vi "integracao_1.03.vi"() -> ()   [LabVIEW 2011]
panel:
  out "Waveform Chart 4":dynamicdata(graph)
  out "Waveform Chart 3":dbl(graph)
  in  "Numeric 7":dbl
  in  "Numeric 6":dbl
  in  "Numeric 5":dbl
  in  "Numeric 4":dbl
  in  "Numeric 3":dbl
  in  "Numeric 2":dbl
  in  "Numeric":dbl
  in  "tail n-1":dbl
  in  "tail":dbl
  out "Integral 2 anter":dbl
  out "Integral 2 n-1":dbl
  out "Area  pico":dbl
  out "tempo 3":dbl
  out "Integral 3":dbl
  out "slope neg n-1":bool
  out "tempo 2":dbl
  out "Integral 2":dbl
  out "slope pos n-1":bool
  in  "picos":dbl
  out "Boolean 4":bool
  out "appended path":path
  out "String":string
  in  "Arquivo de entrada 2":path=path "C:/Works/GC3000/datalog/GC3000"
  out "Array":string[](array[string])
  out "Integral":dbl
  out "pico real":bool
  out "slope negativo":bool
  out "slope positivo":bool
  out "delta tempo menor 0,025":bool
  out "sinal menor que 1":bool
  out "signal 2":dbl
  out "Boolean 3":bool
  out "tempo":dbl
  out "Boolean 2":bool
  out "Waveform Chart 2":dynamicdata(graph)
  out "Boolean":bool
  out "slop curve":dbl
  out "Result":dbl
  out "signal":dbl
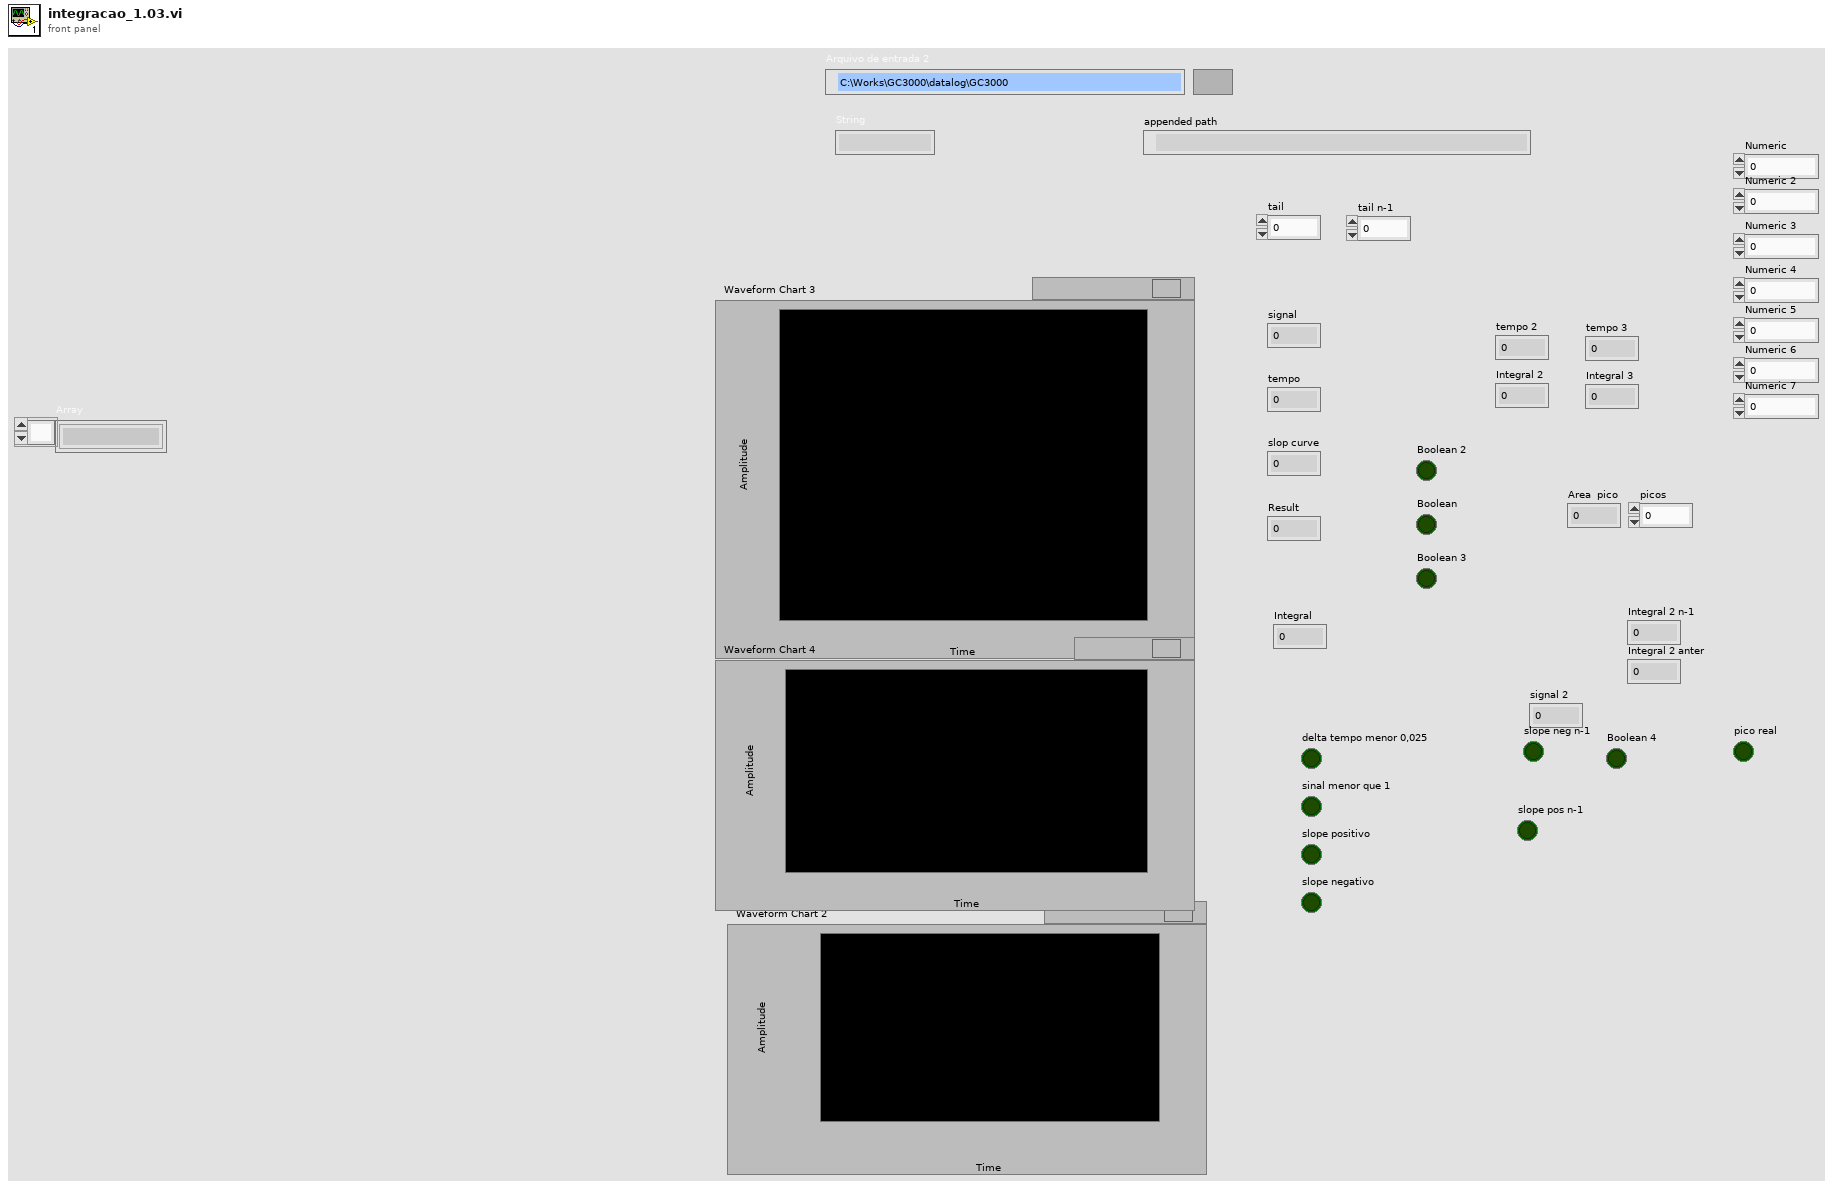
[diagram p1: front panel]
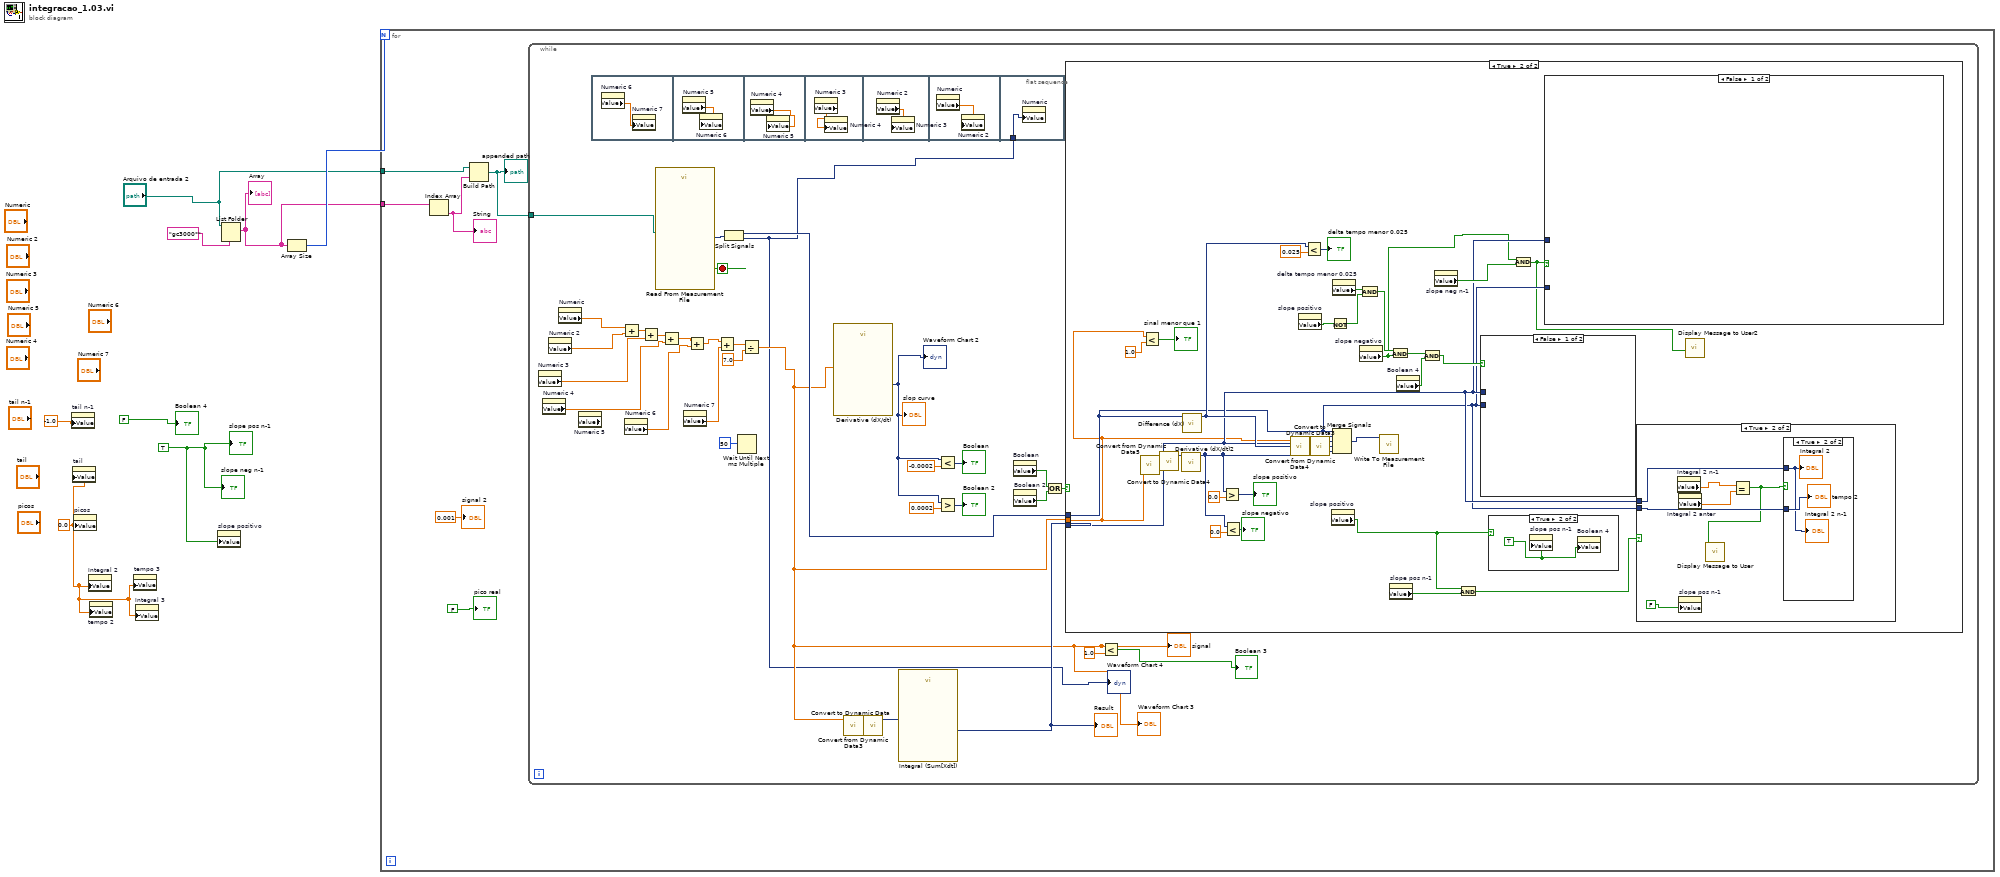
[diagram p0: block diagram]
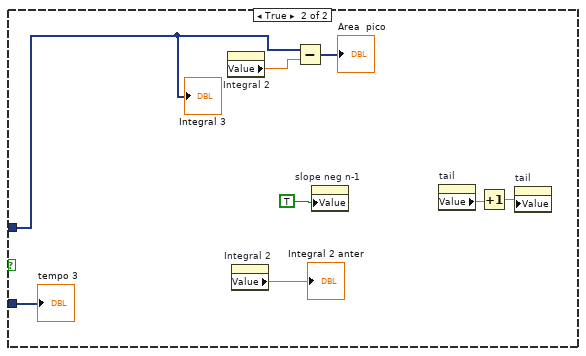
[diagram p3: hidden frame]
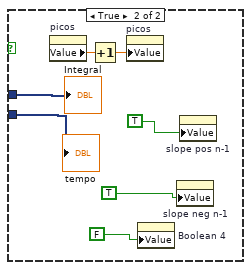
[diagram p7: hidden frame]
diagram:
  w1 = TRUE
  w2 = 0.0 ("picos")
  n1 = property on="tail n-1" class="DigNum (strict)"("Value"=-1.0 ("picos")) -> ()  [unwired: 2 in, 2 out]
  n2 = property on="tail" class="DigNum (strict)"("Value"=w2) -> ()  [unwired: 2 in, 2 out]
  n3 = property on="picos" class="DigNum (strict)"("Value"=w2) -> ()  [unwired: 2 in, 2 out]
  n4 = property on="Integral 2" class="DigNum (strict)"("Value"=w2) -> ()  [unwired: 2 in, 2 out]
  n5 = property on="tempo 2" class="DigNum (strict)"("Value"=w2) -> ()  [unwired: 2 in, 2 out]
  n6 = property on="tempo 3" class="DigNum (strict)"("Value"=w2) -> ()  [unwired: 2 in, 2 out]
  n7 = property on="Integral 3" class="DigNum (strict)"("Value"=w2) -> ()  [unwired: 2 in, 2 out]
  n8 = property on="slope positivo" class="Bool (strict)"("Value"=w1) -> ()  [unwired: 2 in, 2 out]
  n9 = List Folder(path="Arquivo de entrada 2", pattern="gc3000*") -> (filenames=w5:string[])  [unwired: 1 in, 4 out]
  "Array" <- w5
  n10 = Array Size(array=w5) -> (size(s)=w7:i32)
  n11 = for {
    N: w7 -> [_]
    tunnel: "Arquivo de entrada 2" -> [w9]
    tunnel: w5 -> [w11]
    n12 = Index Array(array=w11) -> (element=w12:string)  [unwired: 1 in]
    "String" <- w12
    n13 = Build Path(base path=w9, name or relative path=w12) -> (appended path=w10:path)
    "appended path" <- w10
    n14 = while {
      tunnel: w10 -> [w33]
      stop <- w46 stop-if-true
      n15 = property on="Numeric 3" class="DigNum (strict)"() -> ("Value"=w26:dbl)  [unwired: 2 in, 2 out]
      n16 = property on="Numeric 4" class="DigNum (strict)"() -> ("Value"=w24:dbl)  [unwired: 2 in, 2 out]
      n17 = property on="Numeric 2" class="DigNum (strict)"() -> ("Value"=w27:dbl)  [unwired: 2 in, 2 out]
      n18 = property on="Numeric" class="DigNum (strict)"() -> ("Value"=w29:dbl)  [unwired: 2 in, 2 out]
      n19 = property on="Numeric 5" class="DigNum (strict)" props=["Value"]() -> ()  [unwired: 2 in, 3 out]
      n20 = flat-sequence {
        tunnel: w15 -> [w53]
        frame #0 {
          n21 = property on="Numeric 6" class="DigNum (strict)"() -> ("Value"=w47:dbl)  [unwired: 2 in, 2 out]
          n22 = property on="Numeric 7" class="DigNum (strict)"("Value"=w47) -> ()  [unwired: 2 in, 2 out]
        }
        frame #1 {
          n23 = property on="Numeric 5" class="DigNum (strict)"() -> ("Value"=w48:dbl)  [unwired: 2 in, 2 out]
          n24 = property on="Numeric 6" class="DigNum (strict)"("Value"=w48) -> ()  [unwired: 2 in, 2 out]
        }
        frame #2 {
          n25 = property on="Numeric 4" class="DigNum (strict)"() -> ("Value"=w49:dbl)  [unwired: 2 in, 2 out]
          n26 = property on="Numeric 5" class="DigNum (strict)"("Value"=w49) -> ()  [unwired: 2 in, 2 out]
        }
        frame #3 {
          n27 = property on="Numeric 3" class="DigNum (strict)"() -> ("Value"=w50:dbl)  [unwired: 2 in, 2 out]
          n28 = property on="Numeric 4" class="DigNum (strict)"("Value"=w50) -> ()  [unwired: 2 in, 2 out]
        }
        frame #4 {
          n29 = property on="Numeric 2" class="DigNum (strict)"() -> ("Value"=w51:dbl)  [unwired: 2 in, 2 out]
          n30 = property on="Numeric 3" class="DigNum (strict)"("Value"=w51) -> ()  [unwired: 2 in, 2 out]
        }
        frame #5 {
          n31 = property on="Numeric" class="DigNum (strict)"() -> ("Value"=w52:dbl)  [unwired: 2 in, 2 out]
          n32 = property on="Numeric 2" class="DigNum (strict)"("Value"=w52) -> ()  [unwired: 2 in, 2 out]
        }
        frame #6 {
          n33 = property on="Numeric" class="DigNum (strict)"("Value"=w53) -> ()  [unwired: 2 in, 2 out]
        }
      }
      n34 = Add(x=w29, y=w27) -> (x+y=w28:dbl)
      n35 = property on="Numeric 6" class="DigNum (strict)"() -> ("Value"=w21:dbl)  [unwired: 2 in, 2 out]
      n36 = Add(x=w28, y=w26) -> (x+y=w25:dbl)
      n37 = call "Read From Measurement File"("Filename"=w33) -> ("Signals"=w40:dynamicdata, "EOF?"=w46:bool)  [unwired: 5 in, 4 out]
      n38 = Add(x=w25, y=w24) -> (x+y=w22:dbl)
      n39 = property on="Numeric 7" class="DigNum (strict)"() -> ("Value"=w18:dbl)  [unwired: 2 in, 2 out]
      n40 = Add(x=w22, y=w21) -> (x+y=w19:dbl)
      n41 = Add(x=w19, y=w18) -> (x+y=w17:dbl)
      n42 = Split Signals(w40) -> (w39:dynamicdata, w15:dynamicdata)  [unwired: 2 in]
      "Waveform Chart 4" <- w15
      n43 = Wait Until Next ms Multiple(millisecond multiple=u32 50) -> ()  [unwired: 1 out]
      n44 = Divide(x=w17, y=7.0) -> (x/y=w16:dbl)
      "signal" <- w16
      "Waveform Chart 3" <- w16
      n45 = call "Derivative (dX/dt)"("Signals"=w16) -> ("Result"=w23:dynamicdata)  [unwired: 5 in, 1 out]
      "slop curve" <- w23
      "Waveform Chart 2" <- w23
      n46 = call "Convert from Dynamic Data3"("Dynamic Data Type"=w16) -> ("Array"=w31:dbl[])  [unwired: 3 in]
      n47 = call "Convert to Dynamic Data"("Array"=w31) -> ("Dynamic Data Type"=w32:dynamicdata)  [unwired: 3 in]
      n48 = call "Integral (Sum[Xdt])"("Signals"=w32) -> ("Result"=w35:dynamicdata)  [unwired: 5 in, 1 out]
      "Result" <- w35
      n49 = Less?(x=w23, y=-0.0002) -> (x < y?=→"Boolean":dynamicdata)
      n50 = Greater?(x=w23, y=0.0002) -> (0:→"Boolean 2":dynamicdata)
      n51 = property on="Boolean" class="Bool (strict)"() -> ("Value"=w38:bool)  [unwired: 2 in, 2 out]
      n52 = property on="Boolean 2" class="Bool (strict)"() -> ("Value"=w37:bool)  [unwired: 2 in, 2 out]
      n53 = Or(x=w38, y=w37) -> (x .or. y?=w36:bool)
      n54 = case shown="True" w36 {
        tunnel: w39 -> [_ w63]
        tunnel: w16 -> [_ w54]
        tunnel: w35 -> [_ w64]
        frame False {
        }
        frame True {
          n55 = call "Convert from Dynamic Data5"("Dynamic Data Type"=w54) -> ("Array"=w56:dbl[])  [unwired: 3 in]
          n56 = Less?(x=w54, y=1.0) -> (x < y?=→"sinal menor que 1":bool)
          n57 = call "Convert to Dynamic Data4"("Array"=w56) -> ("Dynamic Data Type"=w58:dynamicdata)  [unwired: 3 in]
          n58 = call "Derivative (dX/dt)2"("Signals"=w58) -> ("Result"=w77:dynamicdata)  [unwired: 5 in, 1 out]
          n59 = call "Difference (dX)"("Signals"=w63) -> ("Result"=w82:dynamicdata)  [unwired: 5 in, 1 out]
          n60 = Greater?(x=w77, y=0.0) -> (0:→"slope positivo":dynamicdata)
          n61 = Less?(x=w77, y=0.0) -> (x < y?=→"slope negativo":dynamicdata)
          n62 = call "Convert from Dynamic Data4"("Dynamic Data Type"=w54) -> ("Array"=w57:dbl[])  [unwired: 3 in]
          n63 = property on="slope positivo" class="Bool (strict)"() -> ("Value"=w73:bool)  [unwired: 2 in, 2 out]
          n64 = Less?(x=w82, y=0.025) -> (x < y?=→"delta tempo menor 0,025":dynamicdata)
          n65 = call "Convert to Dynamic Data3"("Array"=w57) -> ("Dynamic Data Type"=w59:dynamicdata)  [unwired: 3 in]
          n66 = Not(x=w73) -> (.not. x?=w72:bool)
          n67 = property on="slope positivo" class="Bool (strict)"() -> ("Value"=w61:bool)  [unwired: 2 in, 2 out]
          n68 = property on="delta tempo menor 0,025" class="Bool (strict)"() -> ("Value"=w75:bool)  [unwired: 2 in, 2 out]
          n69 = Merge Signals(w63, w59, w64, w82, w77) -> (w84:dynamicdata)
          n70 = property on="slope negativo" class="Bool (strict)"() -> ("Value"=w62:bool)  [unwired: 2 in, 2 out]
          n71 = And(x=w75, y=w72) -> (x .and. y?=w71:bool)
          n72 = call "Write To Measurement File"("Signals"=w84) -> ()  [unwired: 16 in, 3 out]
          n73 = property on="slope pos n-1" class="Bool (strict)"() -> ("Value"=w67:bool)  [unwired: 2 in, 2 out]
          n74 = And(x=w71, y=w62) -> (x .and. y?=w70:bool)
          n75 = property on="Boolean 4" class="Bool (strict)"() -> ("Value"=w68:bool)  [unwired: 2 in, 2 out]
          n76 = And(x=w70, y=w68) -> (x .and. y?=w69:bool)
          n77 = property on="slope neg n-1" class="Bool (strict)"() -> ("Value"=w65:bool)  [unwired: 2 in, 2 out]
          n78 = And(x=w61, y=w67) -> (x .and. y?=w66:bool)
          n79 = case shown="False" w69 {
            tunnel: w64 -> [_ w108]
            tunnel: w63 -> [_ w107]
            frame False {
            }
            frame True {
              n80 = property on="picos" class="DigNum (strict)"() -> ("Value"=w106:dbl)  [unwired: 2 in, 2 out]
              n81 = Increment(x=w106) -> (x+1=w105:dbl)
              n82 = property on="picos" class="DigNum (strict)"("Value"=w105) -> ()  [unwired: 2 in, 2 out]
              n83 = property on="Boolean 4" class="Bool (strict)"("Value"=FALSE) -> ()  [unwired: 2 in, 2 out]
              n84 = property on="slope neg n-1" class="Bool (strict)"("Value"=TRUE) -> ()  [unwired: 2 in, 2 out]
              n85 = property on="slope pos n-1" class="Bool (strict)"("Value"=TRUE) -> ()  [unwired: 2 in, 2 out]
              "Integral" <- w108
              "tempo" <- w107
            }
          }
          n86 = case shown="True" w61 {
            frame False {
            }
            frame True {
              w101 = TRUE
              n87 = property on="slope pos n-1" class="Bool (strict)"("Value"=w101) -> ()  [unwired: 2 in, 2 out]
              n88 = property on="Boolean 4" class="Bool (strict)"("Value"=w101) -> ()  [unwired: 2 in, 2 out]
            }
          }
          n89 = And(x=w62, y=w65) -> (x .and. y?=w60:bool)
          n90 = case shown="False" w60 {
            tunnel: w64 -> [_ w92]
            tunnel: w63 -> [_ w91]
            frame False {
            }
            frame True {
              n91 = property on="Integral 2" class="DigNum (strict)"() -> ("Value"=w89:dbl)  [unwired: 2 in, 2 out]
              n92 = property on="Integral 2" class="DigNum (strict)"() -> ("Value"=→"Integral 2 anter":dbl)  [unwired: 2 in, 2 out]
              n93 = Subtract(x=w92, y=w89) -> (x-y=→"Area  pico":dynamicdata)
              n94 = property on="slope neg n-1" class="Bool (strict)"("Value"=TRUE ("slope neg n-1")) -> ()  [unwired: 2 in, 2 out]
              n95 = property on="tail" class="DigNum (strict)"() -> ("Value"=w85:dbl)  [unwired: 2 in, 2 out]
              n96 = Increment(x=w85) -> (x+1=w86:dbl)
              n97 = property on="tail" class="DigNum (strict)"("Value"=w86) -> ()  [unwired: 2 in, 2 out]
              "Integral 3" <- w92
              "tempo 3" <- w91
            }
          }
          n98 = case shown="True" w66 {
            tunnel: w64 -> [_ w98]
            tunnel: w63 -> [_ w97]
            frame False {
            }
            frame True {
              n99 = property on="Integral 2 n-1" class="DigNum (strict)"() -> ("Value"=w95:dbl)  [unwired: 2 in, 2 out]
              n100 = property on="Integral 2 anter" class="DigNum (strict)"() -> ("Value"=w94:dbl)  [unwired: 2 in, 2 out]
              n101 = property on="slope pos n-1" class="Bool (strict)"("Value"=FALSE) -> ()  [unwired: 2 in, 2 out]
              n102 = Equal?(x=w95, y=w94) -> (x = y?=w93:bool)
              n103 = call "Display Message to User"("Enable"=w93) -> ()  [unwired: 9 in, 2 out]
              n104 = case shown="True" w93 {
                tunnel: w98 -> [_ w99]
                tunnel: w97 -> [_ w100]
                frame False {
                }
                frame True {
                  "Integral 2" <- w99
                  "tempo 2" <- w100
                  "Integral 2 n-1" <- w99
                }
              }
            }
          }
          n105 = call "Display Message to User2"("Enable"=w60) -> ()  [unwired: 9 in, 2 out]
        }
      }
      n106 = Less?(x=w16, y=1.0) -> (x < y?=→"Boolean 3":bool)
    }
    "signal 2" <- 0.001 ("signal 2")
    "pico real" <- FALSE ("pico real")
  }
  "Boolean 4" <- FALSE
  "slope pos n-1" <- w1
  "slope neg n-1" <- w1
